vi "update visited list.vi"(6 "previous node string":string, 8 "edge cost":dbl, 9 "previous node":refnum<data-value>, 10 "current node":refnum<data-value>, 11 "visited list in":variant) -> (0 "path cost":dbl, 1 "replaced":bool, 2 "discarded":bool, 3 "visited list out":variant)   [LabVIEW 2017, in "NI_Robotics_Navigation .lvlib"]
uses:
  <vilib>/robotics/Navigation/NI_Robotics_Navigation .lvlib
  <vilib>/robotics/Navigation/shared/MapNode/AbstractAstarNode/NI_Robotics_AbstractAstarNode.lvclass
  c:/Program Files (x86)/National Instruments/LabVIEW 2017/vi.lib/robotics/Navigation/shared/MapNode/AbstractMapNode/NI_Robotics_AbstractMapNode.lvclass
  <vilib>/robotics/Navigation/Astar/Visited List Element.ctl
  <vilib>/robotics/Navigation/shared/MapNode/AbstractMapNode/NI_Robotics_AbstractMapNode.lvclass
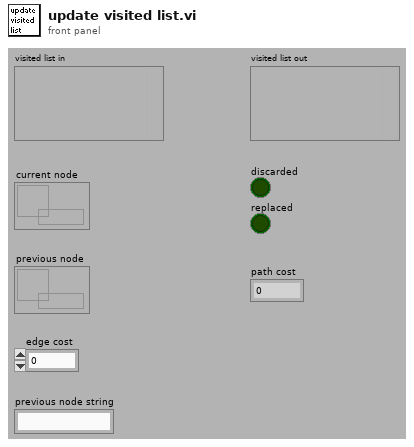
[diagram p1: front panel]
types:
  T1 = typedef "NI_Robotics_Navigation .lvlib/Visited List Element.ctl" = cluster{"Best cost to state":dbl, "Back pointer":refnum<data-value>}
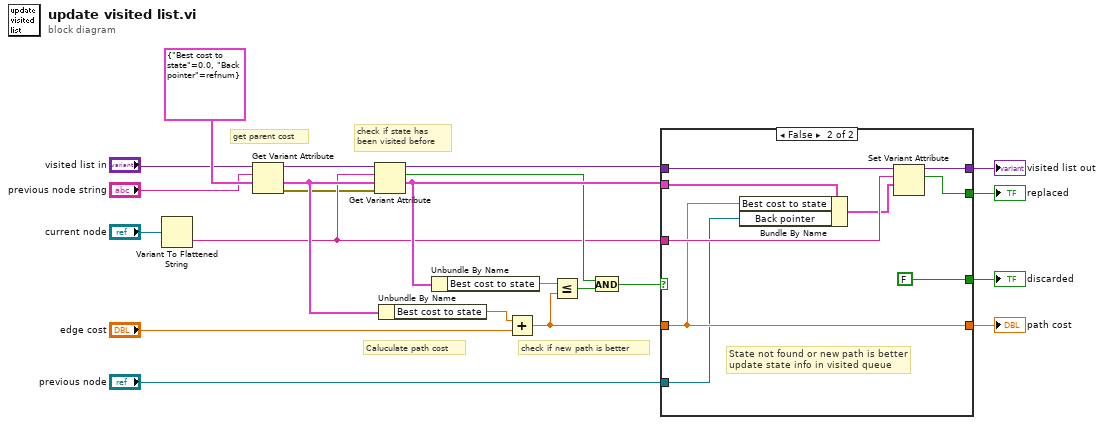
[diagram p0: block diagram]
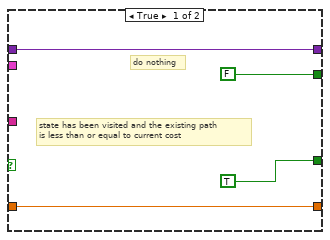
[diagram p2: hidden frame]
diagram:
  # "Caluculate path cost"
  # "get parent cost"
  # "check if new path is better"
  # "check if state has \nbeen visited before"
  n1 = Variant To Flattened String(Variant="current node") -> (data string=w4:string)  [unwired: 1 out]
  n2 = Get Variant Attribute(Variant="visited list in", name="previous node string", default value (empty Variant)=T1 {"Best cost to state"=0.0, "Back pointer"=refnum} ("Visited Element")) -> (duplicate Variant=w11:variant, value=w10:T1, error out=w1:errorcluster)  [unwired: 1 in, 1 out]
  n3 = Get Variant Attribute(Variant=w11, name=w4, default value (empty Variant)=w10, error in=w1) -> (duplicate Variant=w20:variant, found=w17:bool, value=w21:T1)  [unwired: 1 out]
  n4 = Unbundle By Name(w10) -> ("Best cost to state"=w9:dbl)
  n5 = Unbundle By Name(w21) -> ("Best cost to state"=w22:dbl)
  n6 = Add(x=w9, y="edge cost") -> (x+y=w7:dbl)
  n7 = Less Or Equal?(x=w22, y=w7) -> (x <= y?=w19:bool)
  n8 = And(x=w17, y=w19) -> (x .and. y?=w18:bool)
  n9 = case shown="False" w18 {
    tunnel: w21 -> [_ w35]
    tunnel: w20 -> [w26 w34]
    tunnel: [w26 w31] -> w15
    tunnel: w7 -> [w24 w29]
    tunnel: w4 -> [_ w33]
    tunnel: [TRUE FALSE] -> w16
    tunnel: [FALSE ("replaced") w30] -> w14
    tunnel: "previous node" -> [_ w27]
    tunnel: [w24 w29] -> w6
    frame True {
      # "do nothing"
      # "state has been visited and the existing path\nis less than or equal to current cost"
    }
    frame False {
      # "State not found or new path is better\nupdate state info in visited queue"
      n10 = Bundle By Name(cluster=w35, "Best cost to state"=w29, "Back pointer"=w27) -> (w32:T1)
      n11 = Set Variant Attribute(Variant=w34, name=w33, value=w32) -> (Variant out=w31:variant, replaced=w30:bool)  [unwired: 1 in, 1 out]
    }
  }
  "discarded" <- w16
  "visited list out" <- w15
  "replaced" <- w14
  "path cost" <- w6
